vi "conj.vi"(0 "Conj.InitCyc*2^32":u32, 1 "ConjArr":cluster{"Ratio*2^15":u16, "CycleDiff":u64}[](array[cluster])=[{"Ratio*2^15"=0, "CycleDiff"=0}, {"Ratio*2^15"=0, "CycleDiff"=0}, {"Ratio*2^15"=0, "CycleDiff"=0}, {"Ratio*2^15"=0, "CycleDiff"=0}, {"Ratio*2^15"=0, "CycleDiff"=0}, {"Ratio*2^15"=0, "CycleDiff"=0}, {"Ratio*2^15"=0, "CycleDiff"=0}, {"Ratio*2^15"=0, "CycleDiff"=0}, {"Ratio*2^15"=0, "CycleDiff"=0}, {"Ratio*2^15"=0, "CycleDiff"=0}, {"Ratio*2^15"=0, "CycleDiff"=0}, {"Ratio*2^15"=0, "CycleDiff"=0}, {"Ratio*2^15"=0, "CycleDiff"=0}, {"Ratio*2^15"=0, "CycleDiff"=0}, {"Ratio*2^15"=0, "CycleDiff"=0}, {"Ratio*2^15"=0, "CycleDiff"=0}], 2 "Init_strobe":bool, 5 "ConjSize-1":u8, 9 "1/DeCyc*2^8":u32, 11 "RfCyc_in":u64, 12 "Mode":bool=TRUE) -> (3 "LastConj":bool, 4 "ConjIndex":u8, 6 "Initialising?":bool, 8 "chaseCyc":u64, 10 "Not Conj?":bool, 15 "RfCyc_out":u64)   [LabVIEW 2018]
uses:
  <instrlib>/_niInstr/Basic Elements/v1/FPGA/Private/Count Down U16.vi
  <instrlib>/_niInstr/Basic Elements/v1/FPGA/niInstr Basic Elements v1 FPGA.lvlib
panel:
  out "Cross Conj?":bool
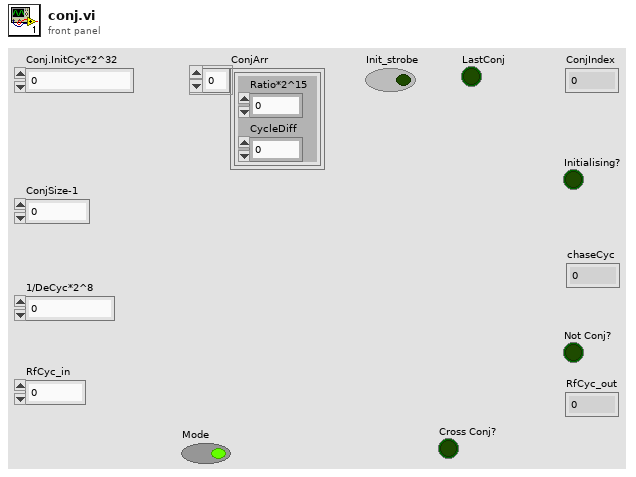
[diagram p1: front panel]
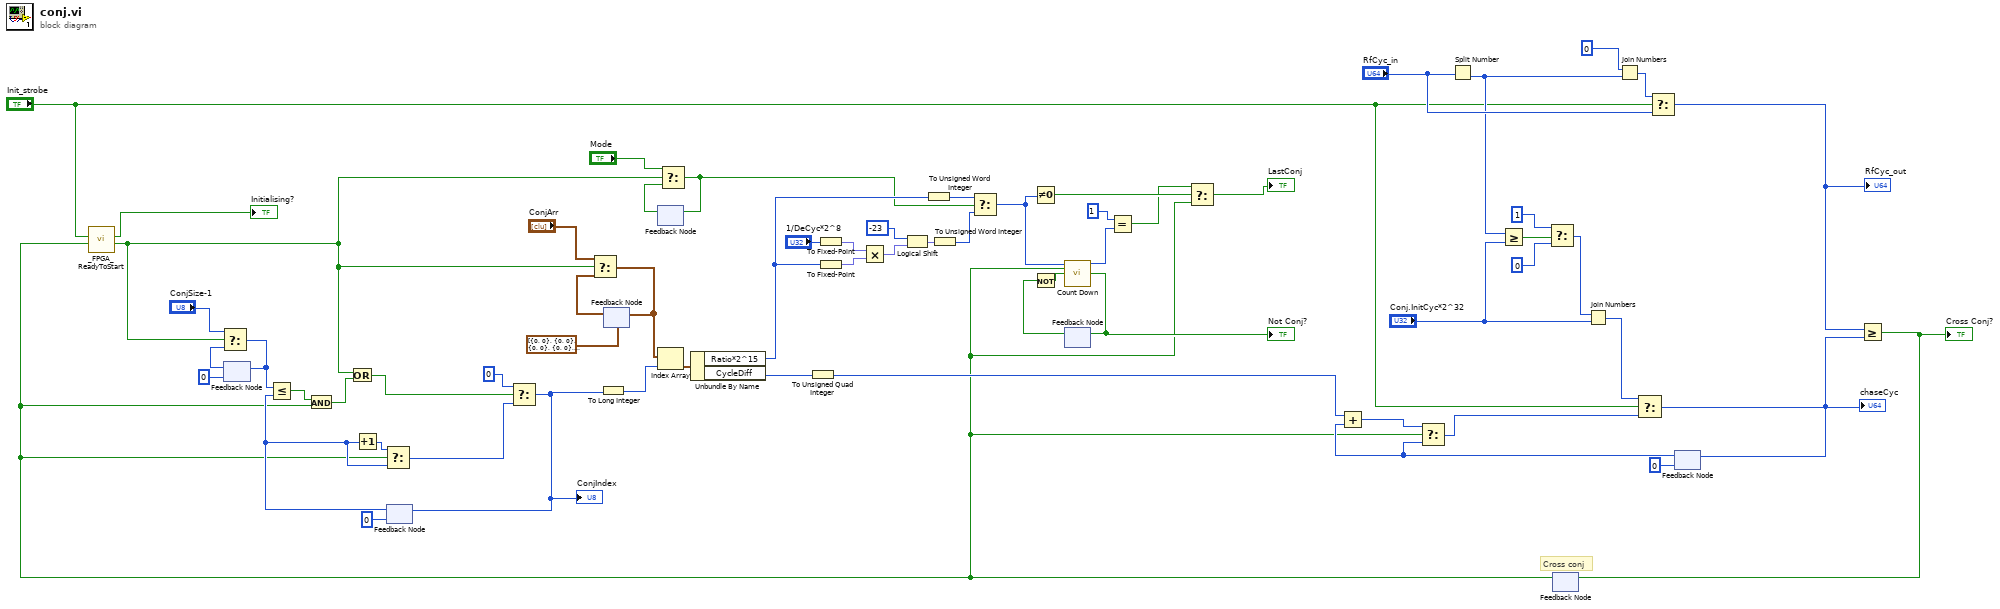
[diagram p0: block diagram]
diagram:
  # "Cross conj"
  n1 = feedback #1(u8 0 ("ConjSize-1")) -> (w36:u8)
  n2 = feedback #2(u8 0) -> (w53:u8)
  n3 = Increment(x=w53) -> (x+1=w54:u8)
  n4 = feedback #3(cluster{"Ratio*2^15":u16, "CycleDiff":u64}[] [{"Ratio*2^15"=0, "CycleDiff"=0}, {"Ratio*2^15"=0, "CycleDiff"=0}, {"Ratio*2^15"=0, "CycleDiff"=0}, {"Ratio*2^15"=0, "CycleDiff"=0}, {"Ratio*2^15"=0, "CycleDiff"=0}, {"Ratio*2^15"=0, "CycleDiff"=0}, {"Ratio*2^15"=0, "CycleDiff"=0}, {"Ratio*2^15"=0, "CycleDiff"=0}, {"Ratio*2^15"=0, "CycleDiff"=0}, {"Ratio*2^15"=0, "CycleDiff"=0}, {"Ratio*2^15"=0, "CycleDiff"=0}, {"Ratio*2^15"=0, "CycleDiff"=0}, {"Ratio*2^15"=0, "CycleDiff"=0}, {"Ratio*2^15"=0, "CycleDiff"=0}, {"Ratio*2^15"=0, "CycleDiff"=0}, {"Ratio*2^15"=0, "CycleDiff"=0}] ("ConjArr")) -> (w49:cluster{"Ratio*2^15":u16, "CycleDiff":u64}[])
  n5 = feedback #4() -> (w7:bool)  [unwired: 1 in]
  n6 = To Fixed-Point(number="1/DeCyc*2^8") -> (fixed-point=w44:fxp<+,32,32>)  [unwired: 1 in]
  n7 = feedback #5() -> (w39:bool)  [unwired: 1 in]
  n8 = Not(x=w39) -> (.not. x?=w40:bool)
  n9 = Split Number(x="RfCyc_in") -> (lo(x)=w33:u32)  [unwired: 1 out]
  n10 = Greater Or Equal?(x=w33, y="Conj.InitCyc*2^32") -> (x >= y?=w31:bool)
  n11 = Select(t=u32 1 ("hi"), s=w31, f=u32 0 ("hi(x)")) -> (s? t:f=w28:u32)
  n12 = feedback #6() -> (w15:bool)  [unwired: 1 in]
  n13 = call "_FPGA_ReadyToStart.vi"("Start_strobe_in"=w15, "Ready_latch_in"="Init_strobe") -> ("Trigger_strobe_out"=w5:bool, "Ready?"=→"Initialising?":bool)  [unwired: 8 in]
  n14 = Select(t="ConjSize-1", s=w5, f=w36) -> (s? t:f=w37:u8)
  n15 = feedback-in #1(w37) -> ()
  n16 = Less Or Equal?(x=w37, y=w53) -> (x <= y?=w56:bool)
  n17 = And(x=w56, y=w15) -> (x .and. y?=w42:bool)
  n18 = Or(x=w5, y=w42) -> (x .or. y?=w34:bool)
  n19 = Select(t=w54, s=w15, f=w53) -> (s? t:f=w51:u8)
  n20 = Select(t=u8 0, s=w34, f=w51) -> (s? t:f=w43:u8)
  "ConjIndex" <- w43
  n21 = feedback-in #2(w43) -> ()
  n22 = Select(t="ConjArr", s=w5, f=w49) -> (s? t:f=w41:cluster{"Ratio*2^15":u16, "CycleDiff":u64}[])
  n23 = To Long Integer(number=w43) -> (32bit integer=w57:i32)
  n24 = feedback-in #3(w41) -> ()
  n25 = Index Array(array=w41, index=w57) -> (element=w58:cluster{"Ratio*2^15":u16, "CycleDiff":u64})
  n26 = Select(t="Mode", s=w5, f=w7) -> (s? t:f=w8:bool)
  n27 = feedback-in #4(w8) -> ()
  n28 = Unbundle By Name(w58) -> ("Ratio*2^15"=w10:u16, "CycleDiff"=w59:u64)
  n29 = To Unsigned Quad Integer(1:w59) -> (0:w35:u64)
  n30 = To Fixed-Point(number=w10) -> (fixed-point=w60:fxp<+,16,16>)  [unwired: 1 in]
  n31 = Multiply(x=w44, y=w60) -> (x*y=w61:fxp<+,48,48>)
  n32 = Logical Shift(y=i16 -23, x=w61) -> (x << y=w63:fxp<+,48,48>)
  n33 = To Unsigned Word Integer(number=w10) -> (unsigned 16bit integer=w13:u16)
  n34 = To Unsigned Word Integer(number=w63) -> (unsigned 16bit integer=w14:u16)
  n35 = Select(t=w13, s=w8, f=w14) -> (s? t:f=w11:u16)
  n36 = Not Equal To 0?(x=w11) -> (x != 0?=w19:bool)
  n37 = call-poly <instrlib>:"Count Down.vi"("count in"=w11, "load"=w15, "decrement"=w40) -> ("count out"=w21:u16, "terminal count"=w16:bool)  [unwired: 11 in]
  "Not Conj?" <- w16
  n38 = feedback-in #5(w16) -> ()
  n39 = Equal?(x=u16 1, y=w21) -> (x = y?=w18:bool)
  n40 = Select(t=w18, s=w19, f=w15) -> (s? t:f=→"LastConj":bool)
  n41 = Join Numbers(hi=w28, lo="Conj.InitCyc*2^32") -> ((hi.lo)=w27:u64)
  n42 = Join Numbers(hi=u32 0 ("hi(x)"), lo=w33) -> ((hi.lo)=w46:u64)
  n43 = Select(t=w46, s="Init_strobe", f="RfCyc_in") -> (s? t:f=w26:u64)
  "RfCyc_out" <- w26
  n44 = feedback #7(u64 0) -> (w50:u64)
  n45 = Add(x=w35, y=w50) -> (x+y=w55:u64)
  n46 = Select(t=w55, s=w15, f=w50) -> (s? t:f=w48:u64)
  n47 = Select(t=w27, s="Init_strobe", f=w48) -> (s? t:f=w1:u64)
  "chaseCyc" <- w1
  n48 = feedback-in #7(w1) -> ()
  n49 = Greater Or Equal?(x=w26, y=w1) -> (x >= y?=w45:bool)
  "Cross Conj?" <- w45
  n50 = feedback-in #6(w45) -> ()
